vi "OAT Easy Resample Spectral Map (Digital Tach).vi"(0 "scaled signal [EU]":waveform(dbl)={"t0"=timestamp(0 s since 1904-01-01), "dt"=0.0, "Y"=[]}, 1 "dB On (T)":bool=TRUE, 7 "digital tach info":T6={"tacho counts"=[], "counter timebase [Hz]"=20000000.0, "counter task type"=enum."event counting", "counter digit (32)"=32}, 9 "pulse/revolution (1)":i32=1, 11 "error in (no error)":errorcluster, 12 "type":T3(ring)=enum."Order-RPM", 13 "window info":T2={"window type"=10, "window length"=2048} {"window type" items=["None"=0, "Hanning"=1, "Hamming"=2, "Blackman-Harris"=3, "Exact Blackman"=4, "Blackman"=5, "Flat Top"=6, "4 Term B-Harris"=7, "7 Term B-Harris"=8, "Low Sidelobe"=9, "Gaussian"=62]; "window length" min=0}) -> (3 "speed profile":T1 {"speed [RPM]" format="%.2f"; "time [s]" format="%.2f"}, 4 "spectral map":dbl[][](array[numeric]) format="%.2f", 6 "scales":T5 {"Y scale"."multiplier" format="%.2f"; "Y scale"."offset" format="%.2f"; "X scale"."multiplier" format="%.2f"; "X scale"."offset" format="%.2f"}, 8 "unit labels":T4, 15 "error out":errorcluster)   [LabVIEW 2017]
doc: "Computes the spectral map of <B>scaled signal [EU]</B> based on the resampling method. You can use this polymorphic VI to obtain a spectral map for an analog tachometer signal or a digital tachometer signal. The data type you wire to the <B>analog tach signal</B> input determines the polymorphic instance to use."
uses:
  <vilib>/addons/Sound and Vibration/Order Analysis/Tach Process/SubVIs/digital tach info.ctl
  <vilib>/addons/Sound and Vibration/Order Analysis/Ref Gabor Order Tracking/window information.ctl
  <vilib>/addons/Sound and Vibration/Order Analysis/Tach Process/SubVIs/speed profile.ctl
  <vilib>/addons/Sound and Vibration/Order Analysis/Tach Process/SoundVib_TachProcess.lvlib
  <vilib>/addons/Sound and Vibration/Order Analysis/Gabor Order Tracking/SoundVib_Gabor.lvlib
panel:
  # "OAT Easy Resample Spectral Map (Digital Tach)"
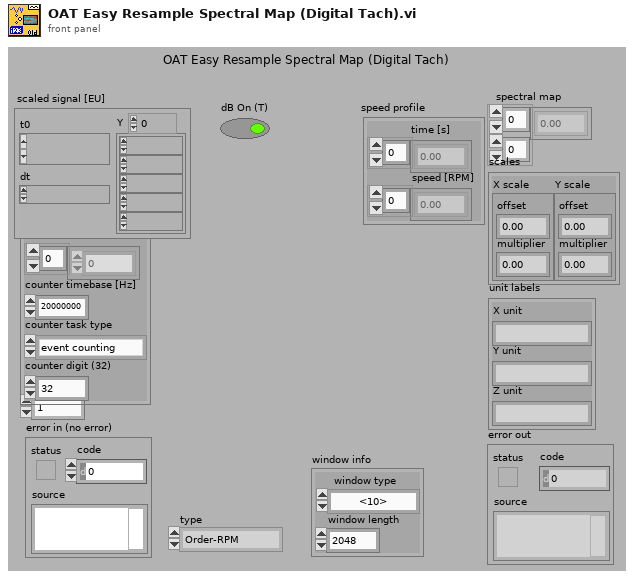
[diagram p1: front panel]
types:
  T1 = typedef "SoundVib_TachProcess.lvlib/speed profile.ctl" = cluster{"time [s]":dbl[], "speed [RPM]":dbl[]}
  T2 = typedef "SoundVib_Gabor.lvlib/window information.ctl" = cluster{"window type":u32, "window length":i32}
  T3 = enum16{"Frequency-Time", "Frequency-RPM", "Order-RPM"}
  T4 = cluster{"X unit":string, "Y unit":string, "Z unit":string}
  T5 = cluster{"X scale":cluster{"offset":dbl, "multiplier":dbl}, "Y scale":cluster{"offset":dbl, "multiplier":dbl}}
  T6 = typedef "SoundVib_TachProcess.lvlib/digital tach info.ctl" = cluster{"tacho counts":i64[], "counter timebase [Hz]":dbl, "counter task type":enum16{"period measurement", "event counting"}, "counter digit (32)":i32}
  T7 = cluster{"type":enum16{"Frequency-Time", "Frequency-RPM", "Order-RPM"}, "range":cluster{"start":dbl, "end":dbl, "step":dbl}}
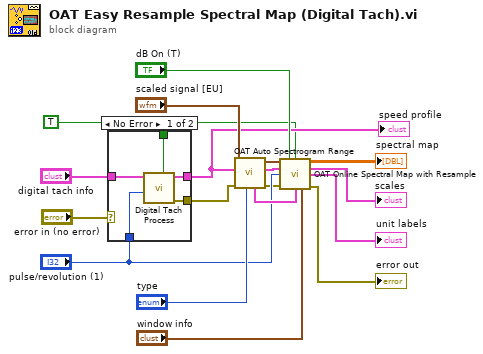
[diagram p0: block diagram]
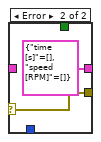
[diagram p2: hidden frame]
diagram:
  w1 = TRUE ("reset? (TRUE)")
  n1 = case shown="No Error" "error in (no error)" {
    selector: "error in (no error)" -> [_ w24]
    tunnel: "digital tach info" -> [w23 _]
    tunnel: "pulse/revolution (1)" -> [w22 _]
    tunnel: [w21 T1 {"time [s]"=[], "speed [RPM]"=[]} ("speed profile")] -> w6
    tunnel: [w20 w24] -> w4
    tunnel: w1 -> [w19 _]
    frame No Error {
      n2 = call <vilib>:"Digital Tach Process.vi"("reset? (True)"=w19, "pulse/revolution (1)"=w22, "digital tach info"=w23) -> ("error out"=w20:errorcluster, "speed profile"=w21:T1)  [unwired: 6 in, 1 out]
    }
    frame Error {
    }
  }
  "speed profile" <- w6
  n3 = call <vilib>:"OAT Auto Spectrogram Range.vi"("type"="type", "error in (no error)"=w4, "speed profile in"=w6, "scaled signal [EU] in"="scaled signal [EU]") -> ("error out"=w3:errorcluster, "speed profile out"=w8:T1, "scaled signal [EU] out"=w12:waveform(dbl), "config"=w9:T7)  [unwired: 4 in]
  n4 = call <vilib>:"OAT Online Spectral Map with Resample.vi"("scaled signal [EU]"=w12, "dB On (T)"="dB On (T)", "reset? (True)"=w1, "speed profile"=w8, "pulse/revolution (1)"="pulse/revolution (1)", "error in (no error)"=w3, "config"=w9, "window info"="window info") -> ("spectral map"=→"spectral map":dbl[][], "scales"=→"scales":T5, "unit labels"=→"unit labels":T4, "error out"=→"error out":errorcluster)  [unwired: 3 in, 1 out]
